vi "ObtainRefLibItems.vi"() -> ()   [LabVIEW 2016]
uses:
  TemplateLibraryItems.ctl
panel:
  out "Array 2":errorcluster[](array[cluster])
  out "Array":string[](array[string])
  out "ItemRefs":refnum<vi>[](array[refnum])
  out "TemplateLibraryItems":T1
  in  "TemplateLibrary":string="LibA.lvlib"
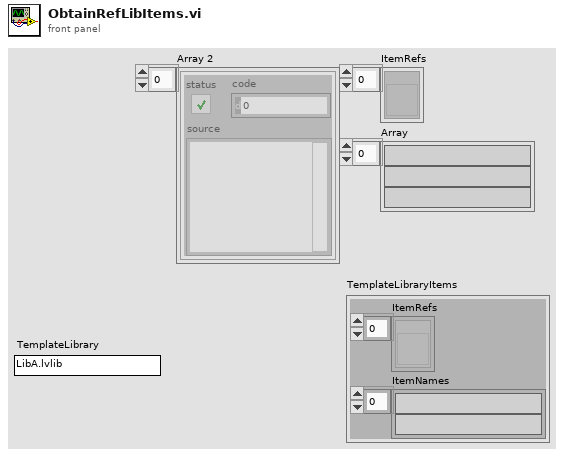
[diagram p1: front panel]
types:
  T1 = typedef "TemplateLibraryItems.ctl" = cluster{"ItemRefs":refnum<vi>[], "ItemNames":string[]}
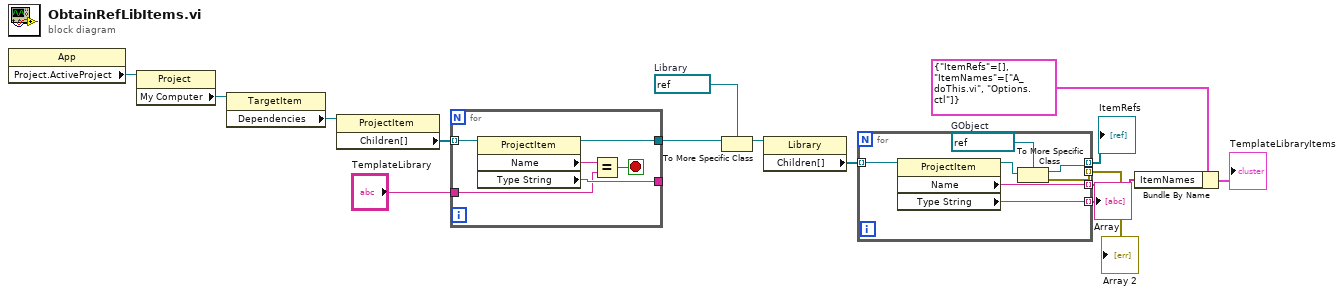
[diagram p0: block diagram]
diagram:
  w9 = refnum<vi> refnum  # Library
  n1 = property class="App"() -> ("Project.ActiveProject"=w15:refnum<vi>)  [unwired: 2 in, 2 out]
  n2 = property class="Project"(reference=w15) -> ("My Computer"=w14:refnum<vi>)  [unwired: 1 in, 2 out]
  n3 = property class="TargetItem"(reference=w14) -> ("Dependencies"=w13:refnum<vi>)  [unwired: 1 in, 2 out]
  n4 = property class="ProjectItem"(reference=w13) -> ("Children[]"=w12:refnum<vi>[])  [unwired: 1 in, 2 out]
  n5 = for {
    tunnel: [w21] -> w10
    tunnel: w12 -> [w19] mode=indexing
    tunnel: [w20] -> _
    tunnel: "TemplateLibrary" -> [w17]
    stop <- w16 stop-if-true
    n6 = property class="ProjectItem"(reference=w19) -> (reference out=w21:refnum<vi>, "Name"=w18:string, "Type String"=w20:string)  [unwired: 1 in, 1 out]
    n7 = Equal?(x=w18, y=w17) -> (x = y?=w16:bool)
  }
  n8 = To More Specific Class(target class=w9, reference=w10) -> (specific class reference=w8:refnum<vi>)  [unwired: 1 in, 1 out]
  n9 = property class="Library"(reference=w8) -> ("Children[]"=w7:refnum<vi>[])  [unwired: 1 in, 2 out]
  n10 = for {
    tunnel: w7 -> [w28] mode=indexing
    tunnel: [w27] -> w5 mode=indexing
    tunnel: [w24] -> w3 mode=indexing
    tunnel: [w23] -> w2 mode=indexing
    tunnel: [w22] -> w1 mode=indexing
    w25 = refnum<vi> refnum  # GObject
    n11 = property class="ProjectItem"(reference=w28) -> (reference out=w26:refnum<vi>, "Name"=w27:string, "Type String"=w23:string)  [unwired: 1 in, 1 out]
    n12 = To More Specific Class(target class=w25, reference=w26) -> (specific class reference=w24:refnum<vi>, error out=w22:errorcluster)  [unwired: 1 in]
  }
  "ItemRefs" <- w3
  "Array" <- w2
  "Array 2" <- w1
  n13 = Bundle By Name(cluster=T1 {"ItemRefs"=[], "ItemNames"=["A_doThis.vi", "Options.ctl"]} ("TemplateLibraryItems"), "ItemNames"=w5) -> (→"TemplateLibraryItems":T1)
